vi "Configure.vi"(8 "error in (no error)":errorcluster, 10 "Msg in":T1, 11 "FakePressureController in":refnum<class "PXIDigitizer.lvclass">) -> (0 "error out":errorcluster, 1 "new command":string, 2 "Msg out":T1, 3 "FakePressureController out":refnum<class "PXIDigitizer.lvclass">)   [LabVIEW 2011, in "PXIDigitizer.lvclass"]
uses:
  PXIDigitizer.lvclass
  DriverMsg.ctl
  PXIDigitizer.lvclass/PXIDigitizer.ctl
  ChannelSettings_TypDef.ctl
  coupling_Enum_TypDef.ctl
  impedance_Enum_TypDEf.ctl
  OnOffTypeDef.ctl
  BaseDriver/BaseDriver.lvclass
panel:
  out "Command":string
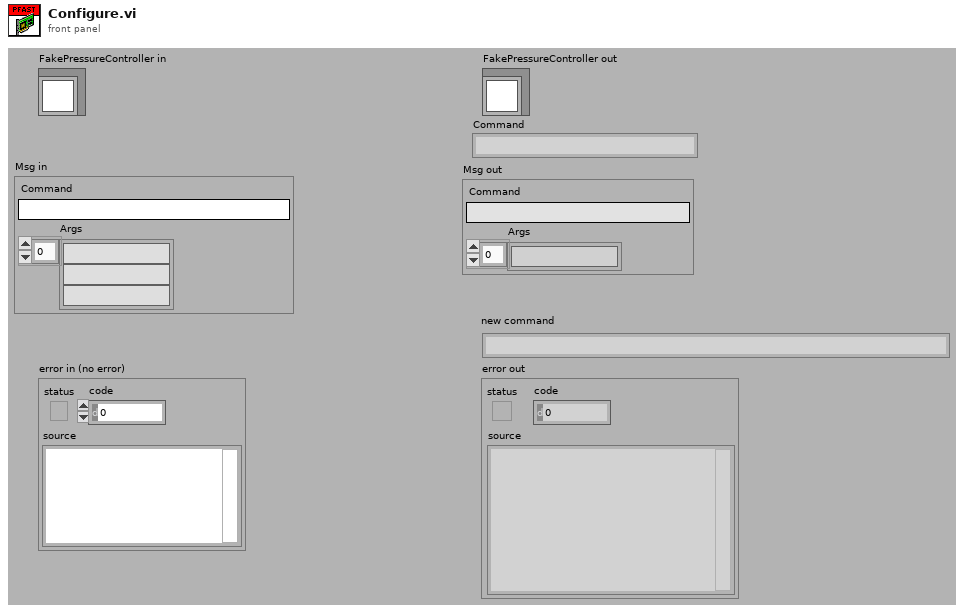
[diagram p1: front panel]
types:
  T1 = typedef "DriverMsg.ctl" = cluster{"Command":string, "Args":string[]}
  T2 = typedef "impedance_Enum_TypDEf.ctl" = enum16{"1 mega ohm", "<NA>", "50 ohms"}
  T3 = typedef "OnOffTypeDef.ctl" = enum16{"off", "on"}
  T4 = typedef "PXIDigitizer.lvclass/settings_TypDef.ctl" = cluster{"resourcename":string, "timeout":T5, "LocalSavingPath":path, "Save":T3, "probeattenuation":cluster{"Channel0":T5, "Channel1":T5, "Channel2":T5, "Channel3":T5, "Channel4":T5, "Channel5":T5, "Channel6":T5, "Channel7":T5}, "channelenabled":T6, "coupling":cluster{"Channel0":T7, "Channel1":T7, "Channel2":T7, "Channel3":T7, "Channel4":T7, "Channel5":T7, "Channel6":T7, "Channel7":T7}, "impedance":cluster{"Channel0":T2, "Channel1":T2, "Channel2":T2, "Channel3":T2, "Channel4":T2, "Channel5":T2, "Channel6":T2, "Channel7":T2}, "Trigger":T8, "Horizontal":T18, "Names":cluster{"Channel0":string, "Channel1":string, "Channel2":string, "Channel3":string, "Channel4":string, "Channel5":string, "Channel6":string, "Channel7":string}, "verticalrange":cluster{"Channel0":T5, "Channel1":T5, "Channel2":T5, "Channel3":T5, "Channel4":T5, "Channel5":T5, "Channel6":T5, "Channel7":T5}, "offset":cluster{"Channel0":T5, "Channel1":T5, "Channel2":T5, "Channel3":T5, "Channel4":T5, "Channel5":T5, "Channel6":T5, "Channel7":T5}, "Number of channels":dbl, "Method":T19, "LinkedChannel":T21}
  T5 = typedef "numericVariable_TypeDef.ctl" = cluster{"Value":dbl, "Min":dbl, "Max":dbl, "StepSize":dbl, "Tolerance":dbl, "valueactual":dbl}
  T6 = typedef "channelenabled_TypDef.ctl" = cluster{"Channel0":T3, "Channel1":T3, "Channel2":T3, "Channel3":T3, "Channel4":T3, "Channel5":T3, "Channel6":T3, "Channel7":T3}
  T7 = typedef "coupling_Enum_TypDef.ctl" = enum16{"AC", "DC", "Ground"}
  T8 = typedef "TriggerSettings_TypDef.ctl" = cluster{"DC Restore":T3, "Polarity":T9, "TV Event":T10, "Coupling":T11, "Slope":T12, "AnalogSource":T13, "Window Mode":T14, "Low Level":dbl, "High Level":dbl, "Hysteresis":dbl, "Delay":dbl, "Holdoff":dbl, "Signal Format":T15, "Mode":T16, "Line Number":i32, "DigitalSource":T17}
  T9 = typedef "Polarity_TypDEf.ctl" = enum16{"Negative", "Positive"}
  T10 = typedef "TVEvent_TypDef.ctl" = enum16{"Field 1", "Field 2", "Any Field", "Any Line", "Line Number"}
  T11 = typedef "coupling_TypDef.ctl" = enum16{"AC", "DC", "HF Reject", "LF Reject", "AC Plus HF Reject"}
  T12 = typedef "positive_negatice2_typDef.ctl" = enum16{"Positive", "Negative"}
  T13 = typedef "TriggerSource_TypDef.ctl" = enum16{"Channel 0", "Channel 1", "External TRIG"}
  T14 = typedef "triggerwindowmode2_TypDef.ctl" = enum16{"Entering", "Leaving"}
  T15 = typedef "SignalFormat_TypDef.ctl" = enum16{"M-NTSC", "B/G-PAL", "SECAM", "M-PAL", "480i/59.94 fps", "480i/60 fps", "480p/59.94 Fps", "480p/60 Fps", "576i/50 fps", "576p/50 Fps", "720p/50 Fps", "720p/59.94 Fps", "720p/60 Fps", "1080i/50 fps", "1080i/59.94 fps", "1080i/60 fps", "1080p/24 Fps"}
  T16 = typedef "mode_TypDef.ctl" = enum32{"Immediate", "Analog Edge", "Analog Window", "Analog Hysteresis", "Video", "Digital Edge"}
  T17 = typedef "Trigger.DigitalSource_TypDEf.ctl" = enum16{"RTSI 0", "RTSI 1", "RTSI 2", "RTSI 3", "RTSI 4", "RTSI 5", "RTSI 6", "PFI 0", "PFI 1", "PFI 2", "PXI Star Trigger"}
  T18 = typedef "horizontal_TypDef.ctl" = cluster{"min sample rate":dbl, "min record length":i32, "actual record length":i32, "actual sample rate":dbl, "Enforce Realtime":T3}
  T19 = typedef "methodCluster_TypDEf.ctl" = cluster{"Analysis1":T20, "Analysis2":T20, "Analysis3":T20, "Analysis4":T20, "Analysis5":T20, "Analysis6":T20, "Analysis7":T20, "Analysis8":T20, "Analysis9":T20, "Analysis10":T20}
  T20 = typedef "method_TypDef.ctl" = enum16{"n/a", "max", "min", "energy"}
  T21 = typedef "LinkedChannelsCluster_TypDef.ctl" = cluster{"Analysis1":T22, "Analysis2":T22, "Analysis3":T22, "Analysis4":T22, "Analysis5":T22, "Analysis6":T22, "Analysis7":T22, "Analysis8":T22, "Analysis9":T22, "Analysis10":T22}
  T22 = typedef "channels_TypDef.ctl" = enum16{"Channel0", "Channel1", "Channel2", "Channel3", "Channel4", "Channel5", "Channel6", "Channel7", "n/a"}
  T23 = typedef "ChannelSettings_TypDef.ctl" = cluster{"verticalrange":dbl, "probeattenuation":dbl, "offset":dbl, "channelenabled":bool, "coupling":T7, "impedance":T2}
  T24 = cluster{"Channel0":string, "Channel1":string, "Channel2":string, "Channel3":string, "Channel4":string, "Channel5":string, "Channel6":string, "Channel7":string}
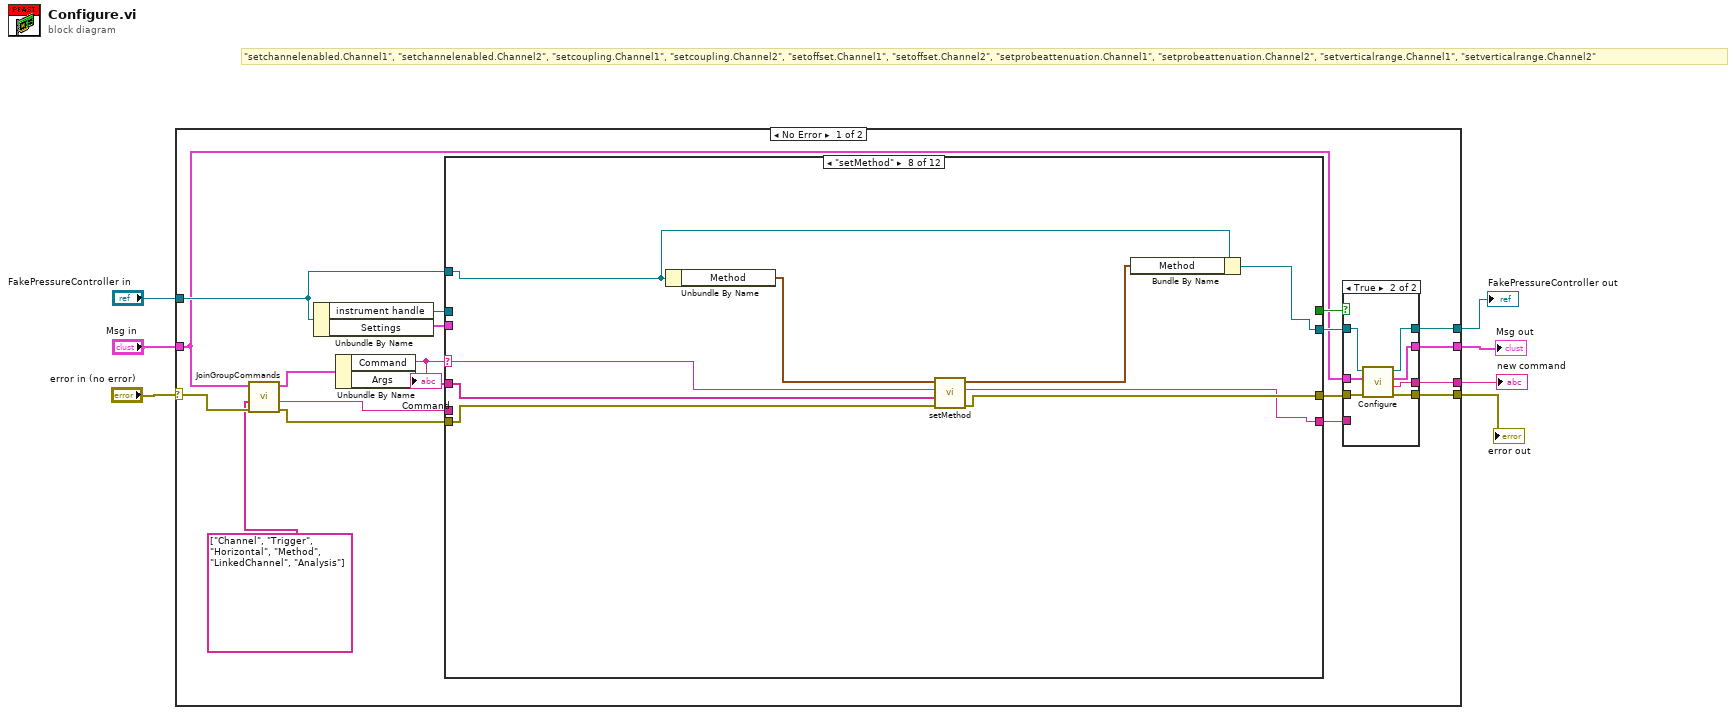
[diagram p0: block diagram]
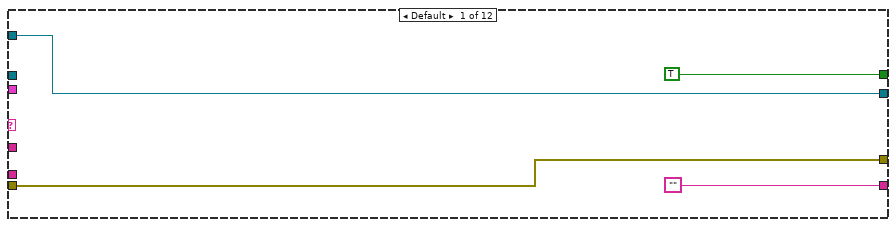
[diagram p3: hidden frame]
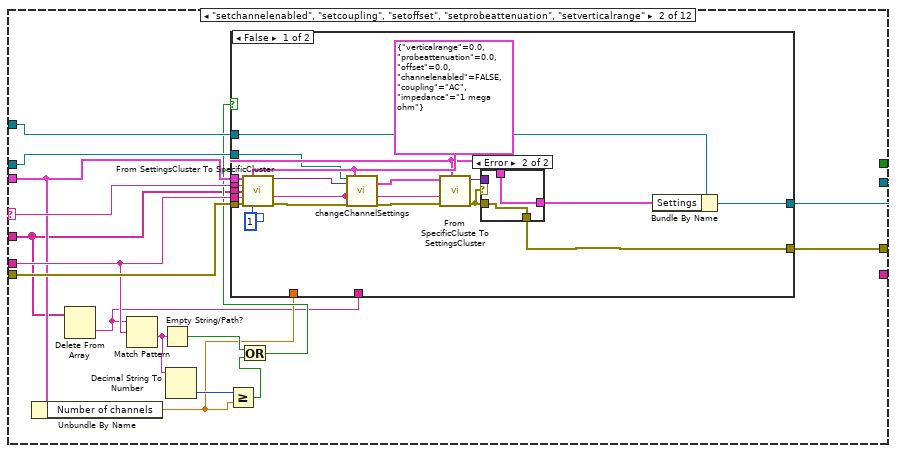
[diagram p4: hidden frame]
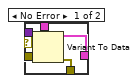
[diagram p5: hidden frame]
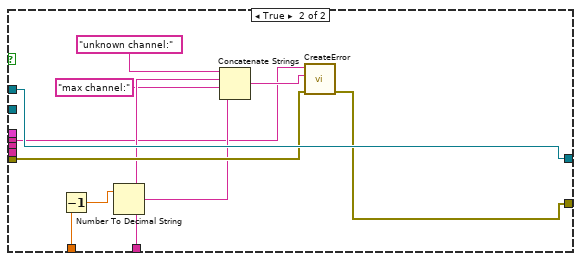
[diagram p6: hidden frame]
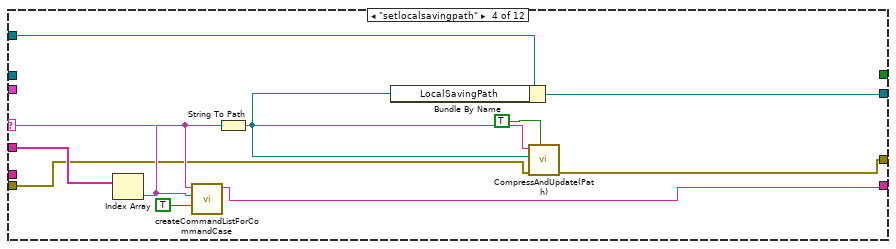
[diagram p8: hidden frame]
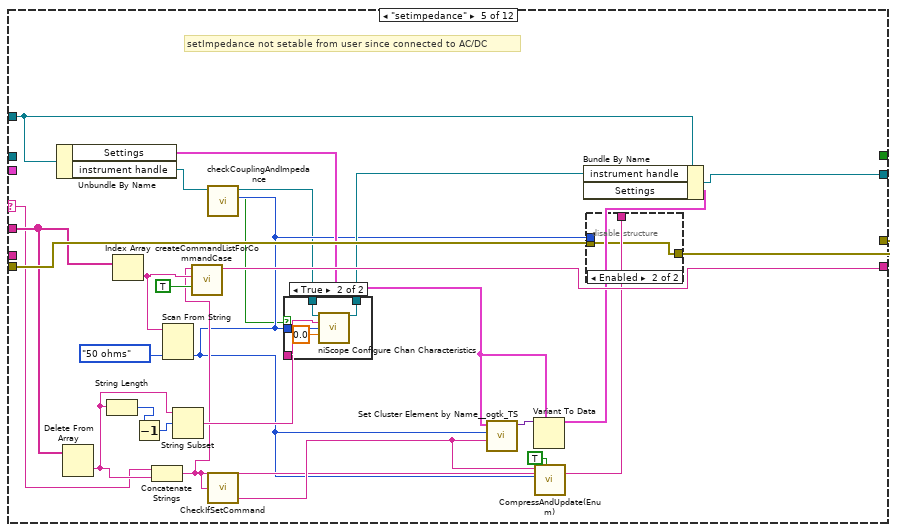
[diagram p9: hidden frame]
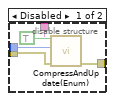
[diagram p11: hidden frame]
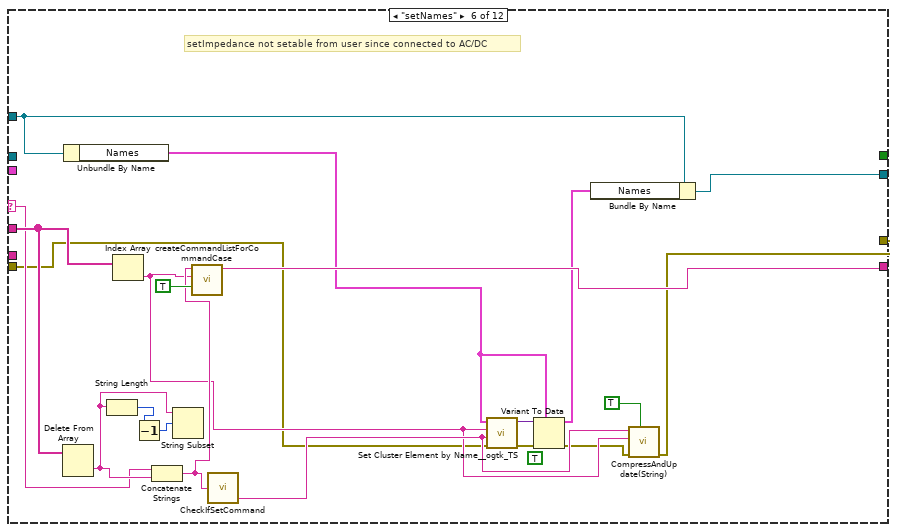
[diagram p12: hidden frame]
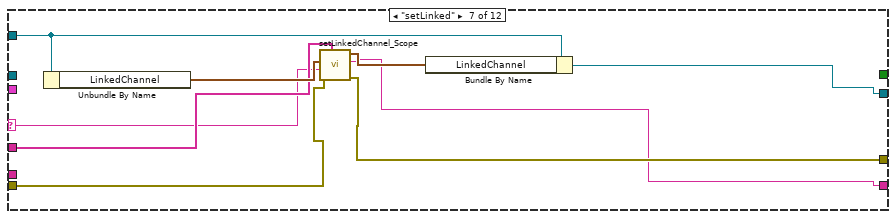
[diagram p13: hidden frame]
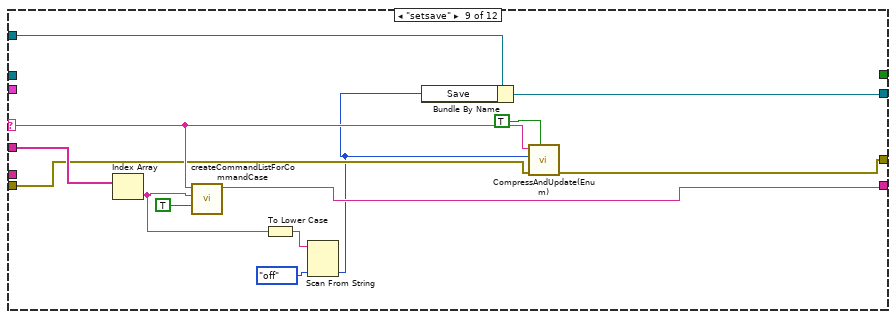
[diagram p14: hidden frame]
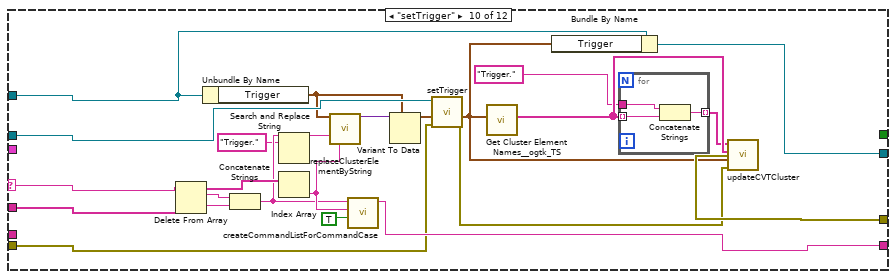
[diagram p15: hidden frame]
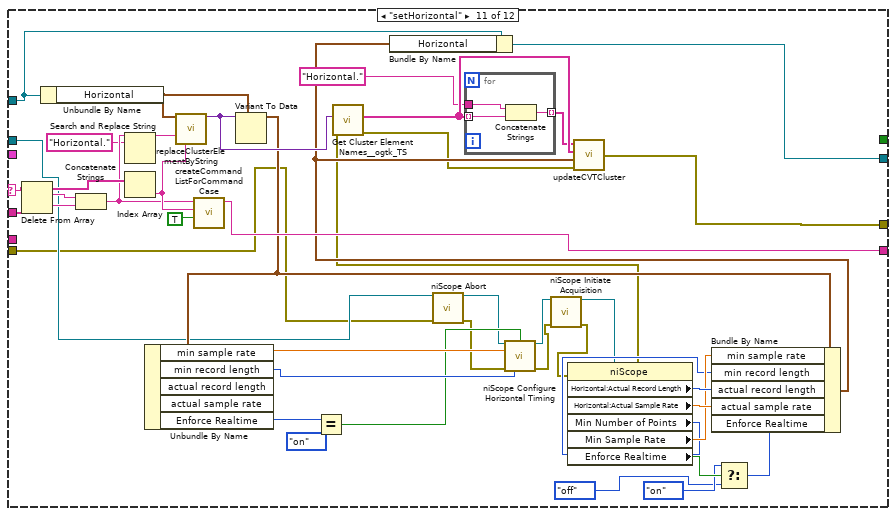
[diagram p16: hidden frame]
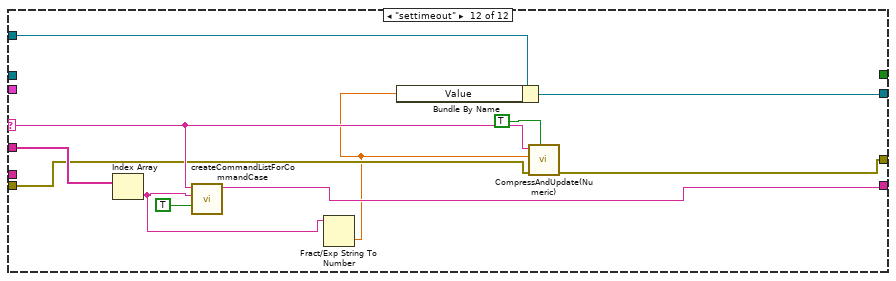
[diagram p17: hidden frame]
diagram:
  # "\"setchannelenabled.Channel1\", \"setchannelenabled.Channel2\", \"setcoupling.Channel1\", \"setcoupling.Channel2\", \"setoffset.Channel1\", \"setoffset.Channel2\", \"setprobeattenuation.Channel1\", \"setprobeattenuation.Channel2\", \"setverticalrange.Channel1\", \"setverticalrange.Channel2\""
  n1 = case shown="No Error" "error in (no error)" {
    selector: "error in (no error)" -> [w13 w279]
    tunnel: "FakePressureController in" -> [w17 w277]
    tunnel: [w25 w277] -> w4
    tunnel: [w23 w279] -> w1
    tunnel: "Msg in" -> [w10 w278]
    tunnel: [w21 w278] -> w3
    tunnel: [w19 _] -> w2
    frame No Error {
      n2 = call "JoinGroupCommands.vi"("error in (no error)"=w13, "Seperator"=string[] ["Channel", "Trigger", "Horizontal", "Method", "LinkedChannel", "Analysis"], "Msg in"=w10) -> ("error out"=w12:errorcluster, "Seperator out"=w9:string, "Msg out"=w11:T1)  [unwired: 6 in]
      n3 = Unbundle By Name(w17) -> ("instrument handle"=w16:refnum<k15>, "Settings"=w15:T4)
      n4 = Unbundle By Name(w11) -> ("Command"=w18:string, "Args"=w14:string[])
      "Command" <- w18
      n5 = case shown="\"setMethod\"" w18 {
        selector: w18 -> [_ w54 _ w102 w113 w153 w169 w179 w191 w214 w260 w272]
        tunnel: w12 -> [w40 w55 w95 w99 w130 w147 w167 w177 w189 w215 w225 w270]
        tunnel: w14 -> [_ w43 _ w105 w121 w158 w170 w178 w193 w213 w259 w274]
        tunnel: w17 -> [w41 w57 w96 w107 w127 w161 w173 w181 w195 w212 w257 w276]
        tunnel: [w41 w56 w96 w97 w128 w162 w172 w174 w187 w211 w221 w268] -> w26
        tunnel: ["" ("Complete") _ _ w103 w131 w163 w165 w175 w192 w217 w261 w273] -> w20
        tunnel: [w40 w52 w95 w98 w129 w146 w166 w176 w188 w210 w248 w269] -> w24
        tunnel: [TRUE _ _ _ _ _ _ _ _ _ _ _] -> w22
        tunnel: w16 -> [_ w53 _ _ _ _ _ _ _ w216 w231 _]
        tunnel: w15 -> [_ w48 _ _ _ _ _ _ _ _ _ _]
        tunnel: w9 -> [_ w51 _ _ _ _ _ _ _ _ _ _]
        frame Default {
        }
        frame "setchannelenabled", "setcoupling", "setoffset", "setprobeattenuation", "setverticalrange" {
          n6 = Unbundle By Name(w48) -> ("Number of channels"=w44:dbl)
          n7 = Delete From Array(array=w43) -> (deleted portion=w42:string)  [unwired: 2 in, 1 out]
          n8 = Match Pattern(string=w42, regular expression=w51) -> (after substring=w50:string)  [unwired: 1 in, 3 out]
          n9 = Empty String/Path?(string/path=w50) -> (empty?=w47:bool)
          n10 = Decimal String To Number(string=w50) -> (number=w49:i32)  [unwired: 2 in, 1 out]
          n11 = Greater Or Equal?(x=w49, y=w44) -> (x >= y?=w46:bool)
          n12 = Or(x=w47, y=w46) -> (x .or. y?=w45:bool)
          n13 = case shown="False" w45 {
            tunnel: w57 -> [w76 w94]
            tunnel: [w75 w94] -> w56
            tunnel: w55 -> [w72 w93]
            tunnel: w54 -> [w66 w84]
            tunnel: w48 -> [w65 _]
            tunnel: w53 -> [w63 _]
            tunnel: [w61 w92] -> w52
            tunnel: w43 -> [w59 _]
            tunnel: w51 -> [w58 _]
            tunnel: w42 -> [_ w90]
            tunnel: w44 -> [_ w88]
            frame False {
              w70 = T23 {"verticalrange"=0.0, "probeattenuation"=0.0, "offset"=0.0, "channelenabled"=FALSE, "coupling"=enum."AC", "impedance"=enum."1 mega ohm"} ("channel settings 2")
              n14 = call "From SettingsCluster To SpecificCluster.vi"("variant  (source)"=w65, "variant (destination)"=w70, "Command"=w66, "Args"=w59, "Seperator (\"\")"=w58, "error in (no error)"=w72, "number of group elements (0)"=1) -> ("variant out"=w69:variant, "Seperator out"=w62:string, "error  out"=w68:errorcluster)  [unwired: 4 in, 2 out]
              n15 = call "changeChannelSettings.vi"("instrument handle"=w63, "variant in"=w69, "channels"=w62, "error in (no error)"=w68, "Channel settings"=w70) -> ("Channel settings out"=w74:T23, "error out"=w71:errorcluster)  [unwired: 12 in, 1 out]
              n16 = call "From SpecificCluste To SettingsCluster.vi"("variant (destination)"=w65, "error in (no error)"=w71, "Seperator (\"\")"=w62, "variant  (source)"=w74) -> ("error  out"=w60:errorcluster, "variant out"=w73:variant)  [unwired: 5 in, 1 out]
              n17 = case shown="Error" w60 {
                tunnel: w73 -> [w81 _]
                tunnel: w60 -> [w80 w82]
                tunnel: [w79 w83] -> w67
                tunnel: w65 -> [w78 w83]
                tunnel: [w77 w82] -> w61
                frame No Error {
                  n18 = Variant To Data(error in=w80, type=w78, Variant=w81) -> (data=w79:T4, error out=w77:errorcluster)
                }
                frame Error {
                }
              }
              n19 = Bundle By Name(cluster=w76, "Settings"=w67) -> (w75:refnum<class "PXIDigitizer.lvclass">)
            }
            frame True {
              n20 = Decrement(x=w88) -> (x-1=w87:dbl)
              n21 = Number To Decimal String(number=w87) -> (decimal integer string=w86:string)  [unwired: 1 in]
              n22 = Concatenate Strings("unknown channel:", w90, "max channel:" ("string"), w86) -> (w85:string)
              n23 = call "CreateError.vi"("user error in"=w93, "error message (\"\")"=w85, "command"=w84) -> ("user error  out"=w92:errorcluster)  [unwired: 8 in]
            }
          }
        }
        frame "Abort" {
        }
        frame "setlocalsavingpath" {
          n24 = Index Array(array=w105) -> (element=w104:string)  [unwired: 1 in]
          n25 = call "createCommandListForCommandCase.vi"("immediate Check (only once)"=TRUE, "setvalue"=w104, "command"=w102) -> ("new commands"=w103:string)  [unwired: 8 in]
          n26 = String To Path(string=w104) -> (path=w101:path)
          n27 = Bundle By Name(cluster=w107, "LocalSavingPath"=w101) -> (w97:refnum<class "PXIDigitizer.lvclass">)
          n28 = call "CompressAndUpdate(Path).vi"("force CVT update (false)"=TRUE, "error in"=w99, "Path"=w101, "command or variable name"=w102) -> ("error out"=w98:errorcluster)  [unwired: 7 in]
        }
        frame "setimpedance" {
          # "setImpedance not setable from user since connected to AC/DC"
          n29 = Unbundle By Name(w127) -> ("Settings"=w117:T4, "instrument handle"=w111:refnum<k15>)
          n30 = Delete From Array(array=w121) -> (deleted portion=w119:string)  [unwired: 2 in, 1 out]
          n31 = String Length(string=w119) -> (length=w124:i32)
          n32 = Index Array(array=w121) -> (element=w126:string)  [unwired: 1 in]
          n33 = Decrement(x=w124) -> (x-1=w123:i32)
          n34 = Concatenate Strings(w113, w119) -> (w112:string)
          n35 = Scan From String(input string=w126, default 1=impedance_Enum_TypDEf."50 ohms" ("Impedance2")) -> (output 1=w110:T2)  [unwired: 3 in, 3 out]
          n36 = String Subset(string=w119, offset (0)=w123) -> (substring=w120:string)  [unwired: 1 in]
          n37 = call "createCommandListForCommandCase.vi"("immediate Check (only once)"=TRUE, "setvalue"=w126, "command"=w112) -> ("new commands"=w131:string)  [unwired: 8 in]
          n38 = call "checkCouplingAndImpedance.vi"("Impedance2"=w110, "IVI Refnum in"=w111) -> ("x .or. y?"=w108:bool, "IVI Refnum out"=w109:refnum<k15>)  [unwired: 8 in]
          n39 = call "CheckIfSetCommand.vi"("Command"=w112) -> ("variable"=w115:string)  [unwired: 2 out]
          n40 = case shown="True" w108 {
            tunnel: [w133 w138] -> w122
            tunnel: w120 -> [_ w137]
            tunnel: w110 -> [_ w136]
            tunnel: w109 -> [w133 w135]
            frame False {
            }
            frame True {
              n41 = call "niScope Configure Chan Characteristics.vi"("instrument handle"=w135, "channels"=w137, "input impedance"=w136, "maximum input frequency"=0.0) -> ("instrument handle out"=w138:refnum<k15>)  [unwired: 1 in, 10 out]
            }
          }
          n42 = call "Set Cluster Element by Name__ogtk_TS.vi"("Element Name (\"\": New Element Data Name)"=w115, "New Element Value"=w110, "Cluster"=w117) -> ("VCluster out"=w118:variant)  [unwired: 6 in, 2 out]
          n43 = Variant To Data(type=w117, Variant=w118) -> (data=w116:T4)  [unwired: 1 in, 1 out]
          n44 = call "CompressAndUpdate(Enum).vi"("force CVT update (false)"=TRUE, "enum variant"=w110, "command or variable name"=w115) -> ()  [unwired: 8 in, 1 out]
          n45 = Bundle By Name(cluster=w127, "instrument handle"=w122, "Settings"=w116) -> (w128:refnum<class "PXIDigitizer.lvclass">)
          n46 = disable-structure shown="Enabled" {
            disable-tunnel: w130 -> [w142 w144]
            disable-tunnel: [w141 w144] -> w129
            disable-tunnel: w112 -> [w140 _]
            disable-tunnel: w110 -> [w139 _]
            frame Disabled {
              n47 = call "CompressAndUpdate(Enum).vi"("force CVT update (false)"=TRUE, "error in"=w142, "enum variant"=w139, "command or variable name"=w140) -> ("error out"=w141:errorcluster)  [unwired: 7 in]
            }
            frame Enabled {
            }
          }
        }
        frame "setNames" {
          (unwired) TRUE ("force CVT update (false)")
          # "setImpedance not setable from user since connected to AC/DC"
          n48 = Delete From Array(array=w158) -> (deleted portion=w157:string)  [unwired: 2 in, 1 out]
          n49 = Unbundle By Name(w161) -> ("Names"=w155:T24)
          n50 = String Length(string=w157) -> (length=w160:i32)
          n51 = Index Array(array=w158) -> (element=w150:string)  [unwired: 1 in]
          n52 = Decrement(x=w160) -> (x-1=w159:i32)
          n53 = Concatenate Strings(w153, w157) -> (w152:string)
          n54 = String Subset(string=w157, offset (0)=w159) -> ()  [unwired: 1 in, 1 out]
          n55 = call "createCommandListForCommandCase.vi"("immediate Check (only once)"=TRUE, "setvalue"=w150, "command"=w152) -> ("new commands"=w163:string)  [unwired: 8 in]
          n56 = call "CheckIfSetCommand.vi"("Command"=w152) -> ("variable"=w151:string)  [unwired: 2 out]
          n57 = call "Set Cluster Element by Name__ogtk_TS.vi"("error in (no error)"=w147, "Element Name (\"\": New Element Data Name)"=w151, "New Element Value"=w150, "Cluster"=w155) -> ("error out"=w148:errorcluster, "VCluster out"=w156:variant)  [unwired: 5 in, 1 out]
          n58 = Variant To Data(error in=w148, type=w155, Variant=w156) -> (data=w154:T24, error out=w149:errorcluster)
          n59 = Bundle By Name(cluster=w161, "Names"=w154) -> (w162:refnum<class "PXIDigitizer.lvclass">)
          n60 = call "CompressAndUpdate(String).vi"("force CVT update (false)"=TRUE, "error in"=w149, "String"=w150, "command or variable name"=w151) -> ("error out"=w146:errorcluster)  [unwired: 7 in]
        }
        frame "setLinked" {
          n61 = Unbundle By Name(w173) -> ("LinkedChannel"=w171:T21)
          n62 = call "setLinkedChannel_Scope.vi"("Args"=w170, "error in (no error)"=w167, "String"=w169, "Settings.LinkedChannel in"=w171) -> ("error out"=w166:errorcluster, "new commands"=w165:string, "Settings.LinkedChannel out"=w168:T21)  [unwired: 5 in]
          n63 = Bundle By Name(cluster=w173, "LinkedChannel"=w168) -> (w172:refnum<class "PXIDigitizer.lvclass">)
        }
        frame "setMethod" {
          n64 = Unbundle By Name(w181) -> ("Method"=w182:T19)
          n65 = call "setMethod.vi"("error in (no error)"=w177, "Args"=w178, "String"=w179, "Settings.Method"=w182) -> ("error out"=w176:errorcluster, "new commands"=w175:string, "Settings.Method"=w180:T19)  [unwired: 5 in]
          n66 = Bundle By Name(cluster=w181, "Method"=w180) -> (w174:refnum<class "PXIDigitizer.lvclass">)
        }
        frame "setsave" {
          n67 = Index Array(array=w193) -> (element=w184:string)  [unwired: 1 in]
          n68 = call "createCommandListForCommandCase.vi"("immediate Check (only once)"=TRUE, "setvalue"=w184, "command"=w191) -> ("new commands"=w192:string)  [unwired: 8 in]
          n69 = To Lower Case(string=w184) -> (all lower case string=w186:string)
          n70 = Scan From String(input string=w186, default 1=OnOffTypeDef."off" ("Settings.Trigger")) -> (output 1=w183:T3)  [unwired: 3 in, 3 out]
          n71 = Bundle By Name(cluster=w195, "Save"=w183) -> (w187:refnum<class "PXIDigitizer.lvclass">)
          n72 = call "CompressAndUpdate(Enum).vi"("force CVT update (false)"=TRUE, "error in"=w189, "enum variant"=w183, "command or variable name"=w191) -> ("error out"=w188:errorcluster)  [unwired: 7 in]
        }
        frame "setTrigger" {
          n73 = Delete From Array(array=w213) -> (deleted portion=w208:string)  [unwired: 2 in, 1 out]
          n74 = Unbundle By Name(w212) -> ("Trigger"=w202:T8)
          n75 = Concatenate Strings(w214, w208) -> (w199:string)
          n76 = Search and Replace String(input string=w199, search string="Trigger.") -> (result string=w198:string)  [unwired: 6 in, 3 out]
          n77 = Index Array(array=w213) -> (element=w200:string)  [unwired: 1 in]
          n78 = call "replaceClusterElementByString.vi"("cluster in"=w202, "Command"=w198, "setvalue"=w200) -> ("cluster out"=w203:variant)  [unwired: 10 in, 2 out]
          n79 = call "createCommandListForCommandCase.vi"("immediate Check (only once)"=TRUE, "setvalue"=w200, "command"=w199) -> ("new commands"=w217:string)  [unwired: 8 in]
          n80 = Variant To Data(type=w202, Variant=w203) -> (data=w201:T8)  [unwired: 1 in, 1 out]
          n81 = call "setTrigger.vi"("error in"=w215, "Trigger Settings"=w201, "instrument handle"=w216) -> ("error out"=w196:errorcluster, "Trigger Settings out"=w207:T8)  [unwired: 6 in, 1 out]
          n82 = call "Get Cluster Element Names__ogtk_TS.vi"("Variant"=w207) -> ("Names (Array)"=w206:string[])  [unwired: 9 in, 1 out]
          n83 = Bundle By Name(cluster=w212, "Trigger"=w207) -> (w211:refnum<class "PXIDigitizer.lvclass">)
          n84 = for {
            tunnel: w206 -> [w220] mode=indexing
            tunnel: "Trigger." -> [w219]
            tunnel: [w218] -> w204 mode=indexing
            n85 = Concatenate Strings(w219, w220) -> (w218:string)
          }
          n86 = call "updateCVTCluster.vi"("error in"=w196, "variant (destination) out"=w207, "Cluster Names"=w206, "CVT Names"=w204) -> ("error out"=w210:errorcluster)
        }
        frame "setHorizontal" {
          n87 = Delete From Array(array=w259) -> (deleted portion=w258:string)  [unwired: 2 in, 1 out]
          n88 = Unbundle By Name(w257) -> ("Horizontal"=w253:T18)
          n89 = Concatenate Strings(w260, w258) -> (w251:string)
          n90 = Search and Replace String(input string=w251, search string="Horizontal.") -> (result string=w250:string)  [unwired: 6 in, 3 out]
          n91 = Index Array(array=w259) -> (element=w252:string)  [unwired: 1 in]
          n92 = call "replaceClusterElementByString.vi"("cluster in"=w253, "Command"=w250, "setvalue"=w252) -> ("cluster out"=w247:variant)  [unwired: 10 in, 2 out]
          n93 = call "createCommandListForCommandCase.vi"("immediate Check (only once)"=TRUE, "setvalue"=w252, "command"=w251) -> ("new commands"=w261:string)  [unwired: 8 in]
          n94 = Variant To Data(type=w253, Variant=w247) -> (data=w244:T18)  [unwired: 1 in, 1 out]
          n95 = Unbundle By Name(w244) -> ("min sample rate"=w246:dbl, "min record length"=w245:i32, "Enforce Realtime"=w238:T3)  [unwired: 2 out]
          n96 = Equal?(x=w238, y=OnOffTypeDef."on" ("Enforce Realtime")) -> (x = y?=w236:bool)
          n97 = call "niScope Abort.vi"("instrument handle"=w231, "error in"=w225) -> ("instrument handle out"=w230:refnum<k15>, "error out"=w226:errorcluster)  [unwired: 12 in]
          n98 = call "niScope Configure Horizontal Timing.vi"("instrument handle"=w230, "enforce realtime"=w236, "min sample rate"=w246, "error in"=w226, "min record length"=w245) -> ("instrument handle out"=w229:refnum<k15>, "error out"=w227:errorcluster)  [unwired: 9 in]
          n99 = call "niScope Initiate Acquisition.vi"("instrument handle"=w229, "error in"=w227) -> ("instrument handle out"=w228:refnum<k15>, "error out"=w223:errorcluster)  [unwired: 12 in]
          n100 = property class="niScope"(reference=w228, error in=w223) -> (error out=w222:errorcluster, "Horizontal:Actual Record Length"=w243:i32, "Horizontal:Actual Sample Rate"=w242:dbl, "Min Number of Points"=w240:i32, "Min Sample Rate"=w241:dbl, "Enforce Realtime"=w235:bool)  [unwired: 1 out]
          n101 = call "Get Cluster Element Names__ogtk_TS.vi"("error in (no error)"=w222, "Variant"=w247) -> ("error out"=w224:errorcluster, "Names (Array)"=w256:string[])  [unwired: 8 in]
          n102 = for {
            tunnel: w256 -> [w265] mode=indexing
            tunnel: "Horizontal." -> [w264]
            tunnel: [w263] -> w254 mode=indexing
            n103 = Concatenate Strings(w264, w265) -> (w263:string)
          }
          n104 = Select(t=OnOffTypeDef."on" ("Enforce Realtime"), s=w235, f=OnOffTypeDef."off" ("Enforce Realtime")) -> (s? t:f=w232:T3)
          n105 = Bundle By Name(cluster=w244, "min sample rate"=w241, "min record length"=w240, "actual record length"=w243, "actual sample rate"=w242, "Enforce Realtime"=w232) -> (w239:T18)
          n106 = Bundle By Name(cluster=w257, "Horizontal"=w239) -> (w221:refnum<class "PXIDigitizer.lvclass">)
          n107 = call "updateCVTCluster.vi"("error in"=w224, "variant (destination) out"=w239, "Cluster Names"=w256, "CVT Names"=w254) -> ("error out"=w248:errorcluster)
        }
        frame "settimeout" {
          n108 = Index Array(array=w274) -> (element=w267:string)  [unwired: 1 in]
          n109 = call "createCommandListForCommandCase.vi"("immediate Check (only once)"=TRUE, "setvalue"=w267, "command"=w272) -> ("new commands"=w273:string)  [unwired: 8 in]
          n110 = Fract/Exp String To Number(string=w267) -> (number=w266:dbl)  [unwired: 3 in, 1 out]
          n111 = Bundle By Name(cluster=w276, "Value"=w266) -> (w268:refnum<class "PXIDigitizer.lvclass">)
          n112 = call "CompressAndUpdate(Numeric).vi"("force CVT update (false)"=TRUE, "error in"=w270, "Numeric"=w266, "command or variable name"=w272) -> ("error out"=w269:errorcluster)  [unwired: 7 in]
        }
      }
      n113 = case shown="True" w22 {
        tunnel: w26 -> [w28 w37]
        tunnel: [w28 w36] -> w25
        tunnel: [w29 w35] -> w19
        tunnel: w24 -> [w27 w34]
        tunnel: [w27 w33] -> w23
        tunnel: w10 -> [w30 w32]
        tunnel: [w30 w31] -> w21
        tunnel: w20 -> [w29 _]
        frame False {
        }
        frame True {
          n114 = call-parent "Configure.vi"("error in (no error)"=w34, "Msg in"=w32, "BaseDriver in"=w37) -> ("error out"=w33:errorcluster, "new command"=w35:string, "Msg out"=w31:T1, "BaseDriver out"=w36:refnum<class "PXIDigitizer.lvclass">)  [unwired: 5 in]
        }
      }
    }
    frame Error {
    }
  }
  "error out" <- w1
  "FakePressureController out" <- w4
  "new command" <- w2
  "Msg out" <- w3
